vi "Teleop.vi"(10 "Match Info":T1={"Autonomous Elapsed Seconds"=0.0, "TeleOp Elapsed Seconds"=0.0, "Disabled Elapsed Seconds"=0.0, "Visited Autonomous"=FALSE, "Visited TeleOp"=FALSE, "Visited Disabled"=FALSE, "Autonomous Settings"={"Autonomous Style"=enum."Independent", "VI Refnum"=refnum}}, 11 "Call Context":T2) -> ()   [LabVIEW 2011]
doc: "This VI is called for each TeleOp packet received from the DS where the robot is not disabled. It is often used to read from the joysticks and update I/O or to update setpoints for timed control loops. It should complete and return within 20 milliseconds or it may miss DS packets."
uses:
  <vilib>/Rock Robotics/WPI/DriverStation/WPI_DriverStationDerivedRobotMode.ctl
  <vilib>/Rock Robotics/WPI/DriverStation/WPI_DriverStationMatch Info.ctl
  Robot Global Data.vi
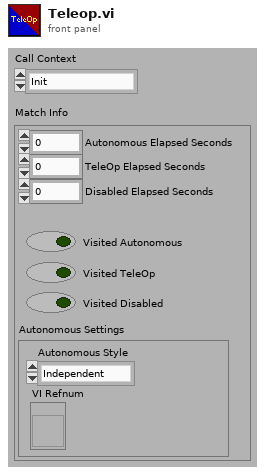
[diagram p1: front panel]
types:
  T1 = typedef "WPI_DriverStationMatch Info.ctl" = cluster{"Autonomous Elapsed Seconds":dbl, "TeleOp Elapsed Seconds":dbl, "Disabled Elapsed Seconds":dbl, "Visited Autonomous":bool, "Visited TeleOp":bool, "Visited Disabled":bool, "Autonomous Settings":cluster{"Autonomous Style":enum16{"Iterative", "Independent"}, "VI Refnum":refnum<vi>}}
  T2 = typedef "WPI_DriverStationDerivedRobotMode.ctl" = enum16{"Init", "Execute", "Stop"}
  T3 = typedef "WPI_JoystickDevRef.ctl" = cluster{"Device":T4}
  T4 = typedef "WPI_JoystickDeviceEnum.ctl" = enum16{"USB 1", "USB 2", "USB 3", "USB 4", "Kinect 1", "Kinect 2"}
  T5 = typedef "WPI_JoystickButtonState.ctl" = cluster{"Button 1":bool, "Button 2":bool, "Button 3":bool, "Button 4":bool, "Button 5":bool, "Button 6":bool, "Button 7":bool, "Button 8":bool, "Button 9":bool, "Button 10":bool, "Button 11":bool, "Button 12":bool}
  T6 = cluster{"axis 1 (x)":dbl, "axis 2 (y)":dbl, "axis 3 (throttle)":dbl, "axis 4":dbl, "axis 5":dbl, "axis 6":dbl}
  T7 = typedef "WPI_AnalogChannelDevRef.ctl" = cluster{"DevStatus":errorcluster, "Analog Module":T8, "Analog Channel":T9}
  T8 = typedef "FPGA_TypedefAnalogModule.ctl" = enum16{"Analog Module 1", "Analog Module 2"}
  T9 = typedef "FPGA_AIChannel.ctl" = enum8{"AI 1", "AI 2", "AI 3", "AI 4", "AI 5", "AI 6", "AI 7", "AI 8", "Invalid"}
  T10 = typedef "WPI_MotorControlDeviceRef.ctl" = cluster{"DeviceStatus":errorcluster, "Type":enum16{"PWM", "CAN"}, "PWM":cluster{"Digital Module":T11, "PWM Channel":T12, "DeadBand":T13}, "CAN":cluster{"Device Number":u8, "Control Mode":T14, "Semaphore":T15, "Max Vout":dbl}, "Invert":bool, "TransformRef":T16, "InvTransformRef":T16}
  T11 = typedef "FPGA_TypedefDigitalModule.ctl" = enum16{"Digital Module 1", "Digital Module 2"}
  T12 = typedef "FPGA_DIOPWMChannel.ctl" = enum8{"PWM 1", "PWM 2", "PWM 3", "PWM 4", "PWM 5", "PWM 6", "PWM 7", "PWM 8", "PWM 9", "PWM 10", "Invalid"}
  T13 = typedef "WPI_PWMDeadband.ctl" = cluster{"Name":string, "maxPositivePwm":i32, "minPositivePwm":i32, "centerPwm":i32, "maxNegativePwm":i32, "minNegativePwm":i32, "angularRange":u16}
  T14 = typedef "WPI_CANJaguar_ControlMode.ctl" = enum8{"Percent VBus", "Current", "Speed", "Position", "Voltage"}
  T15 = typedef "Semaphore RefNum" = refnum<k1>
  T16 = typedef "WPI_PWMTransform_ConPane.ctl" = refnum<vi>
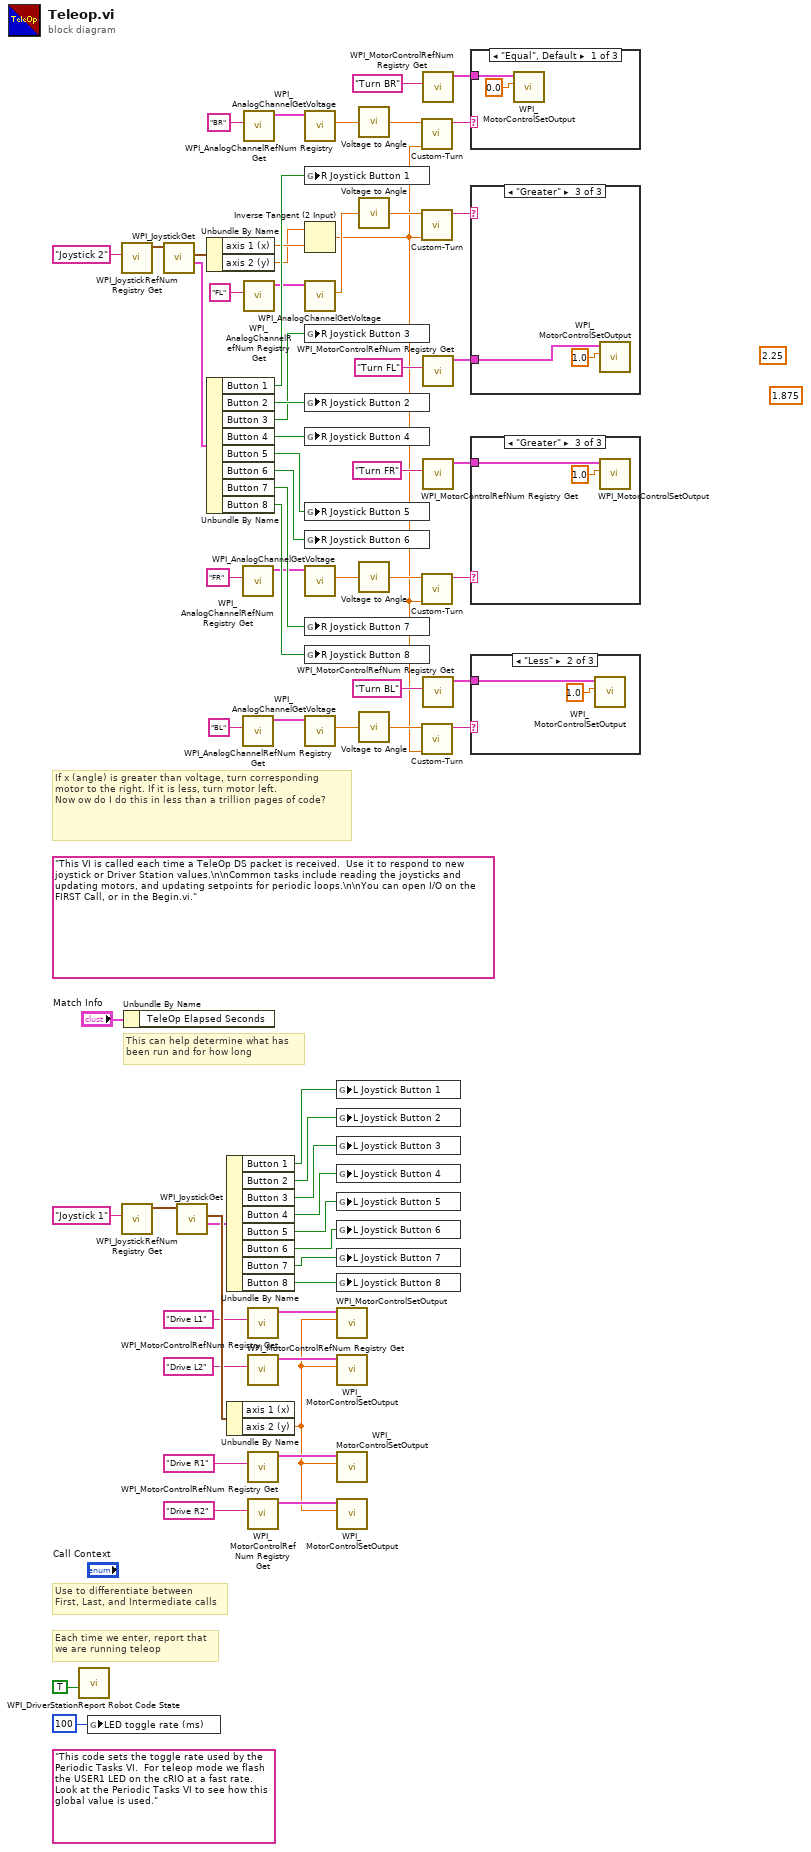
[diagram p0: block diagram]
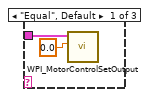
[diagram p2: hidden frame]
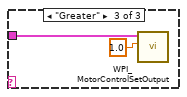
[diagram p3: hidden frame]
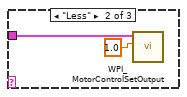
[diagram p4: hidden frame]
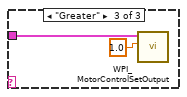
[diagram p5: hidden frame]
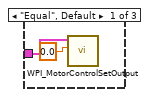
[diagram p6: hidden frame]
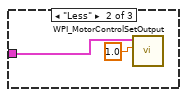
[diagram p7: hidden frame]
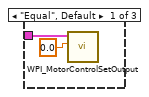
[diagram p8: hidden frame]
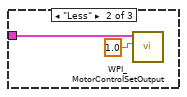
[diagram p9: hidden frame]
diagram:
  (unwired) 1.875
  (unwired) 2.25
  (unwired) "This code sets the toggle rate used by the Periodic Tasks VI.  For teleop mode we flash the USER1 LED on the cRIO at a fast rate.  Look at the Periodic Tasks VI to see how this global value is used."
  (unwired) "This VI is called each time a TeleOp DS packet is received.  Use it to respond to new joystick or Driver Station values.\n\nCommon tasks include reading the joysticks and updating motors, and updating setpoints for periodic loops.\n\nYou can open I/O on the FIRST Call, or in the Begin.vi."
  # "If x (angle) is greater than voltage, turn corresponding motor to the right. If it is less, turn motor left.\nNow ow do I do this in less than a trillion pages of code?"
  # "Each time we enter, report that\nwe are running teleop"
  # "Use to differentiate between\nFirst, Last, and Intermediate calls"
  # "This can help determine what has\nbeen run and for how long"
  n1 = call <vilib>:"WPI_DriverStationReport Robot Code State.vi"("TeleOp"=TRUE ("Autonomous")) -> ()  [unwired: 10 in, 1 out]
  n2 = global write "Robot Global Data.vi" "LED toggle rate (ms)"(u32 100 ("LED ms toggle rate")) -> ()
  n3 = call <vilib>:"WPI_JoystickRefNum Registry Get.vi"("refnum name"="Joystick 2") -> ("JoystickDevRef"=w59:T3)  [unwired: 1 in, 9 out]
  n4 = call <vilib>:"WPI_JoystickRefNum Registry Get.vi"("refnum name"="Joystick 1") -> ("JoystickDevRef"=w64:T3)  [unwired: 1 in, 9 out]
  n5 = Unbundle By Name("Match Info") -> ()  [unwired: 1 out]
  n6 = call <vilib>:"WPI_JoystickGet.vi"("JoystickDevRef"=w59) -> ("Buttons"=w58:T5, "Axes"=w61:T6)  [unwired: 1 in, 4 out]
  n7 = call <vilib>:"WPI_JoystickGet.vi"("JoystickDevRef"=w64) -> ("Buttons"=w57:T5, "Axes"=w66:T6)  [unwired: 1 in, 4 out]
  n8 = Unbundle By Name(w61) -> ("axis 1 (x)"=w40:dbl, "axis 2 (y)"=w39:dbl)
  n9 = Unbundle By Name(w58) -> ("Button 1"=w48:bool, "Button 2"=w47:bool, "Button 3"=w46:bool, "Button 4"=w45:bool, "Button 5"=w44:bool, "Button 6"=w43:bool, "Button 7"=w42:bool, "Button 8"=w41:bool)
  n10 = Unbundle By Name(w57) -> ("Button 1"=w56:bool, "Button 2"=w55:bool, "Button 3"=w54:bool, "Button 4"=w53:bool, "Button 5"=w52:bool, "Button 6"=w51:bool, "Button 7"=w50:bool, "Button 8"=w49:bool)
  n11 = Unbundle By Name(w66) -> ("axis 2 (y)"=w18:dbl)  [unwired: 1 out]
  n12 = call <vilib>:"WPI_AnalogChannelRefNum Registry Get.vi"("refnum name"="FR") -> ("AIDeviceRef"=w32:T7)  [unwired: 9 in, 1 out]
  n13 = call <vilib>:"WPI_AnalogChannelRefNum Registry Get.vi"("refnum name"="BL") -> ("AIDeviceRef"=w34:T7)  [unwired: 9 in, 1 out]
  n14 = call <vilib>:"WPI_AnalogChannelRefNum Registry Get.vi"("refnum name"="BR") -> ("AIDeviceRef"=w36:T7)  [unwired: 9 in, 1 out]
  n15 = call <vilib>:"WPI_AnalogChannelRefNum Registry Get.vi"("refnum name"="FL") -> ("AIDeviceRef"=w38:T7)  [unwired: 9 in, 1 out]
  n16 = call <vilib>:"WPI_MotorControlRefNum Registry Get.vi"("refnum name"="Drive L1") -> ("MotorControlDevRef"=w22:T10)  [unwired: 9 in, 1 out]
  n17 = call <vilib>:"WPI_MotorControlRefNum Registry Get.vi"("refnum name"="Drive L2") -> ("MotorControlDevRef"=w21:T10)  [unwired: 9 in, 1 out]
  n18 = call <vilib>:"WPI_MotorControlRefNum Registry Get.vi"("refnum name"="Drive R1") -> ("MotorControlDevRef"=w20:T10)  [unwired: 9 in, 1 out]
  n19 = call <vilib>:"WPI_MotorControlRefNum Registry Get.vi"("refnum name"="Drive R2") -> ("MotorControlDevRef"=w19:T10)  [unwired: 9 in, 1 out]
  n20 = call <vilib>:"WPI_AnalogChannelGetVoltage.vi"("AIDeviceRef"=w36) -> ("Voltage"=w7:dbl)  [unwired: 8 in, 2 out]
  n21 = global write "Robot Global Data.vi" "R Joystick Button 1"(w48) -> ()
  n22 = Inverse Tangent (2 Input)(1:w40, 2:w39) -> (0:w1:dbl)
  n23 = call <vilib>:"WPI_AnalogChannelGetVoltage.vi"("AIDeviceRef"=w38) -> ("Voltage"=w9:dbl)  [unwired: 8 in, 2 out]
  n24 = global write "Robot Global Data.vi" "R Joystick Button 3"(w46) -> ()
  n25 = global write "Robot Global Data.vi" "R Joystick Button 2"(w47) -> ()
  n26 = global write "Robot Global Data.vi" "R Joystick Button 4"(w45) -> ()
  n27 = global write "Robot Global Data.vi" "R Joystick Button 5"(w44) -> ()
  n28 = global write "Robot Global Data.vi" "R Joystick Button 6"(w43) -> ()
  n29 = call <vilib>:"WPI_AnalogChannelGetVoltage.vi"("AIDeviceRef"=w32) -> ("Voltage"=w3:dbl)  [unwired: 8 in, 2 out]
  n30 = global write "Robot Global Data.vi" "R Joystick Button 7"(w42) -> ()
  n31 = global write "Robot Global Data.vi" "R Joystick Button 8"(w41) -> ()
  n32 = call <vilib>:"WPI_AnalogChannelGetVoltage.vi"("AIDeviceRef"=w34) -> ("Voltage"=w5:dbl)  [unwired: 8 in, 2 out]
  n33 = global write "Robot Global Data.vi" "L Joystick Button 1"(w56) -> ()
  n34 = global write "Robot Global Data.vi" "L Joystick Button 2"(w55) -> ()
  n35 = global write "Robot Global Data.vi" "L Joystick Button 3"(w54) -> ()
  n36 = global write "Robot Global Data.vi" "L Joystick Button 4"(w53) -> ()
  n37 = global write "Robot Global Data.vi" "L Joystick Button 5"(w52) -> ()
  n38 = global write "Robot Global Data.vi" "L Joystick Button 6"(w51) -> ()
  n39 = global write "Robot Global Data.vi" "L Joystick Button 7"(w50) -> ()
  n40 = global write "Robot Global Data.vi" "L Joystick Button 8"(w49) -> ()
  n41 = call <vilib>:"WPI_MotorControlSetOutput.vi"("Output"=w18, "MotorControlDevRef"=w22) -> ()  [unwired: 8 in, 2 out]
  n42 = call <vilib>:"WPI_MotorControlSetOutput.vi"("Output"=w18, "MotorControlDevRef"=w21) -> ()  [unwired: 8 in, 2 out]
  n43 = call <vilib>:"WPI_MotorControlSetOutput.vi"("Output"=w18, "MotorControlDevRef"=w20) -> ()  [unwired: 8 in, 2 out]
  n44 = call <vilib>:"WPI_MotorControlSetOutput.vi"("Output"=w18, "MotorControlDevRef"=w19) -> ()  [unwired: 8 in, 2 out]
  n45 = call "Voltage to Angle.vi"("Numeric"=w7) -> ("Numeric 2"=w6:dbl)  [unwired: 14 in]
  n46 = call "Voltage to Angle.vi"("Numeric"=w9) -> ("Numeric 2"=w8:dbl)  [unwired: 14 in]
  n47 = call "Voltage to Angle.vi"("Numeric"=w3) -> ("Numeric 2"=w2:dbl)  [unwired: 14 in]
  n48 = call "Voltage to Angle.vi"("Numeric"=w5) -> ("Numeric 2"=w4:dbl)  [unwired: 14 in]
  n49 = call "Custom-Turn.vi"("Wanted Angle"=w1, "Wheel Angle"=w6) -> ("Mode"=w13:string)  [unwired: 9 in]
  n50 = call "Custom-Turn.vi"("Wanted Angle"=w1, "Wheel Angle"=w8) -> ("Mode"=w15:string)  [unwired: 9 in]
  n51 = call "Custom-Turn.vi"("Wanted Angle"=w1, "Wheel Angle"=w2) -> ("Mode"=w17:string)  [unwired: 9 in]
  n52 = call "Custom-Turn.vi"("Wanted Angle"=w1, "Wheel Angle"=w4) -> ("Mode"=w11:string)  [unwired: 9 in]
  n53 = call <vilib>:"WPI_MotorControlRefNum Registry Get.vi"("refnum name"="Turn BR") -> ("MotorControlDevRef"=w12:T10)  [unwired: 9 in, 1 out]
  n54 = call <vilib>:"WPI_MotorControlRefNum Registry Get.vi"("refnum name"="Turn FL") -> ("MotorControlDevRef"=w14:T10)  [unwired: 9 in, 1 out]
  n55 = call <vilib>:"WPI_MotorControlRefNum Registry Get.vi"("refnum name"="Turn FR") -> ("MotorControlDevRef"=w16:T10)  [unwired: 9 in, 1 out]
  n56 = call <vilib>:"WPI_MotorControlRefNum Registry Get.vi"("refnum name"="Turn BL") -> ("MotorControlDevRef"=w10:T10)  [unwired: 9 in, 1 out]
  n57 = case shown="\"Equal\", Default" w13 {
    tunnel: w12 -> [w68 w70 w72]
    frame "Equal", Default {
      n58 = call <vilib>:"WPI_MotorControlSetOutput.vi"("Output"=0.0, "MotorControlDevRef"=w68) -> ()  [unwired: 8 in, 2 out]
    }
    frame "Less" {
      n59 = call <vilib>:"WPI_MotorControlSetOutput.vi"("Output"=1.0, "MotorControlDevRef"=w70) -> ()  [unwired: 8 in, 2 out]
    }
    frame "Greater" {
      n60 = call <vilib>:"WPI_MotorControlSetOutput.vi"("Output"=1.0, "MotorControlDevRef"=w72) -> ()  [unwired: 8 in, 2 out]
    }
  }
  n61 = case shown="\"Greater\"" w15 {
    tunnel: w14 -> [w74 w76 w78]
    frame "Equal", Default {
      n62 = call <vilib>:"WPI_MotorControlSetOutput.vi"("Output"=0.0, "MotorControlDevRef"=w74) -> ()  [unwired: 8 in, 2 out]
    }
    frame "Less" {
      n63 = call <vilib>:"WPI_MotorControlSetOutput.vi"("Output"=1.0, "MotorControlDevRef"=w76) -> ()  [unwired: 8 in, 2 out]
    }
    frame "Greater" {
      n64 = call <vilib>:"WPI_MotorControlSetOutput.vi"("Output"=1.0, "MotorControlDevRef"=w78) -> ()  [unwired: 8 in, 2 out]
    }
  }
  n65 = case shown="\"Greater\"" w17 {
    tunnel: w16 -> [w80 w82 w85]
    frame "Equal", Default {
      n66 = call <vilib>:"WPI_MotorControlSetOutput.vi"("Output"=0.0, "MotorControlDevRef"=w80) -> ()  [unwired: 8 in, 2 out]
    }
    frame "Less" {
      n67 = call <vilib>:"WPI_MotorControlSetOutput.vi"("Output"=1.0, "MotorControlDevRef"=w82) -> ()  [unwired: 8 in, 2 out]
    }
    frame "Greater" {
      n68 = call <vilib>:"WPI_MotorControlSetOutput.vi"("Output"=1.0, "MotorControlDevRef"=w85) -> ()  [unwired: 8 in, 2 out]
    }
  }
  n69 = case shown="\"Less\"" w11 {
    tunnel: w10 -> [w86 w88 w90]
    frame "Equal", Default {
      n70 = call <vilib>:"WPI_MotorControlSetOutput.vi"("Output"=0.0, "MotorControlDevRef"=w86) -> ()  [unwired: 8 in, 2 out]
    }
    frame "Less" {
      n71 = call <vilib>:"WPI_MotorControlSetOutput.vi"("Output"=1.0, "MotorControlDevRef"=w88) -> ()  [unwired: 8 in, 2 out]
    }
    frame "Greater" {
      n72 = call <vilib>:"WPI_MotorControlSetOutput.vi"("Output"=1.0, "MotorControlDevRef"=w90) -> ()  [unwired: 8 in, 2 out]
    }
  }
